vi "Finish.vi"   [LabVIEW 2012]
doc: "This VI is called just before exiting. It is expected to close I/O refnum, save collected data, etc."
uses:
  <vilib>/Rock Robotics/WPI/Joystick/WPI_JoystickGetSetRefNum.vi
  <vilib>/Rock Robotics/WPI/RobotDrive/WPI_RobotDriveGetSetRefNum.vi
types:
  T1 = typedef "WPI_CameraDevRef.ctl" = cluster{"Camera Address":string, "CameraStatus":errorcluster, "Acquire Image Notifier":refnum<notifier>}
  T2 = typedef "WPI_JoystickDevRef.ctl" = cluster{"Device":T3}
  T3 = typedef "WPI_JoystickDeviceEnum.ctl" = enum16{"USB 1", "USB 2", "USB 3", "USB 4", "Kinect 1", "Kinect 2"}
  T4 = typedef "WPI_RobotDriveDevRef.ctl" = cluster{"DevStatus":errorcluster, "Motors[]":T5[], "Square Inputs":bool, "Max Output":dbl, "Isochronous":bool}
  T5 = typedef "WPI_MotorControlDeviceRef.ctl" = cluster{"DeviceStatus":errorcluster, "Type":enum16{"PWM", "CAN"}, "PWM":cluster{"Digital Module":T6, "PWM Channel":T7, "DeadBand":T8}, "CAN":cluster{"Device Number":u8, "Control Mode":T9, "Semaphore":T10, "Max Vout":dbl}, "Invert":bool, "TransformRef":T11, "InvTransformRef":T11}
  T6 = typedef "FPGA_TypedefDigitalModule.ctl" = enum16{"Digital Module 1", "Digital Module 2"}
  T7 = typedef "FPGA_DIOPWMChannel.ctl" = enum8{"PWM 1", "PWM 2", "PWM 3", "PWM 4", "PWM 5", "PWM 6", "PWM 7", "PWM 8", "PWM 9", "PWM 10", "Invalid"}
  T8 = typedef "WPI_PWMDeadband.ctl" = cluster{"Name":string, "maxPositivePwm":i32, "minPositivePwm":i32, "centerPwm":i32, "maxNegativePwm":i32, "minNegativePwm":i32, "angularRange":u16}
  T9 = typedef "WPI_CANJaguar_ControlMode.ctl" = enum8{"Percent VBus", "Current", "Speed", "Position", "Voltage"}
  T10 = typedef "Semaphore RefNum" = refnum<k1>
  T11 = typedef "WPI_PWMTransform_ConPane.ctl" = refnum<vi>
  T12 = typedef "WPI_RelayDevRef.ctl" = cluster{"DevStatus":errorcluster, "Relay Channel":T13, "Digital Module":T6, "Relay Direction":T14}
  T13 = typedef "FPGA_DIORelayChannel.ctl" = enum8{"Relay 1", "Relay 2", "Relay 3", "Relay 4", "Relay 5", "Relay 6", "Relay 7", "Relay 8", "Invalid"}
  T14 = typedef "WPI_RelayDirection.ctl" = enum16{"Both directions", "Forward only", "Reverse only"}
  T15 = typedef "WPI_ServoDeviceRef.ctl" = cluster{"DeviceStatus":errorcluster, "Digital Module":T6, "PWM Channel":T7, "DeadBand":T8}
  T16 = typedef "WPI_I2CDevRef.ctl" = cluster{"DevStatus":errorcluster, "Digital Module":T6, "Device Address":u8}
  T17 = typedef "WPI_EncoderDevRef.ctl" = cluster{"DevStatus":errorcluster, "EncoderIndex":T18, "CounterIndex":T19, "DistancePerCount":dbl, "Decoding Type":T20}
  T18 = typedef "FPGA_EncoderIdx.ctl" = enum8{"Enc 0", "Enc 1", "Enc 2", "Enc 3", "Invalid"}
  T19 = typedef "FPGA_CounterCtrSystemIndex.ctl" = enum8{"Ctr 0", "Ctr 1", "Ctr 2", "Ctr 3", "Ctr 4", "Ctr 5", "Ctr 6", "Ctr 7", "Invalid"}
  T20 = typedef "WPI_EncoderType.ctl" = enum16{"1x", "2x", "4x"}
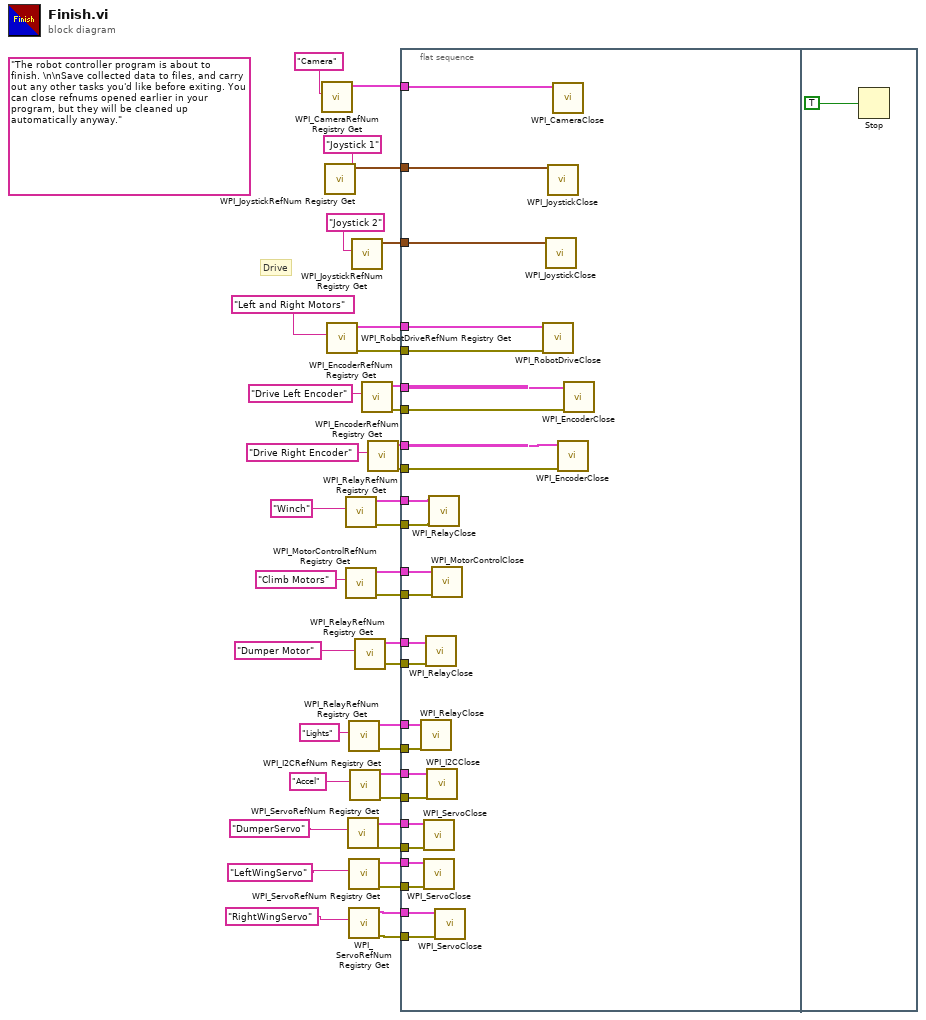
[diagram p0: block diagram]
diagram:
  (unwired) "The robot controller program is about to finish. \n\nSave collected data to files, and carry out any other tasks you'd like before exiting. You can close refnums opened earlier in your program, but they will be cleaned up automatically anyway."
  # "Drive"
  n1 = call <vilib>:"WPI_CameraRefNum Registry Get.vi"("refnum name"="Camera") -> ("CameraDevRef"=w35:T1)  [unwired: 1 in, 9 out]
  n2 = call <vilib>:"WPI_JoystickRefNum Registry Get.vi"("refnum name"="Joystick 1") -> ("JoystickDevRef"=w36:T2)  [unwired: 1 in, 9 out]
  n3 = call <vilib>:"WPI_RobotDriveRefNum Registry Get.vi"("refnum name"="Left and Right Motors") -> ("error out"=w10:errorcluster, "RobotDriveDevRef"=w37:T4)  [unwired: 1 in, 8 out]
  n4 = call <vilib>:"WPI_RelayRefNum Registry Get.vi"("refnum name"="Winch") -> ("error out"=w23:errorcluster, "RelayDevRef"=w24:T12)  [unwired: 9 in]
  n5 = call <vilib>:"WPI_MotorControlRefNum Registry Get.vi"("refnum name"="Climb Motors") -> ("error out"=w21:errorcluster, "MotorControlDevRef"=w22:T5)  [unwired: 9 in]
  n6 = call <vilib>:"WPI_ServoRefNum Registry Get.vi"("refnum name"="DumperServo") -> ("error out"=w4:errorcluster, "ServoDeviceRef"=w5:T15)  [unwired: 9 in]
  n7 = call <vilib>:"WPI_RelayRefNum Registry Get.vi"("refnum name"="Lights") -> ("error out"=w15:errorcluster, "RelayDevRef"=w16:T12)  [unwired: 9 in]
  n8 = call <vilib>:"WPI_ServoRefNum Registry Get.vi"("refnum name"="LeftWingServo") -> ("error out"=w7:errorcluster, "ServoDeviceRef"=w6:T15)  [unwired: 9 in]
  n9 = call <vilib>:"WPI_ServoRefNum Registry Get.vi"("refnum name"="RightWingServo") -> ("error out"=w8:errorcluster, "ServoDeviceRef"=w9:T15)  [unwired: 9 in]
  n10 = call <vilib>:"WPI_I2CRefNum Registry Get.vi"("refnum name"="Accel") -> ("error out"=w11:errorcluster, "I2CDevRef"=w12:T16)  [unwired: 9 in]
  n11 = call <vilib>:"WPI_JoystickRefNum Registry Get.vi"("refnum name"="Joystick 2") -> ("JoystickDevRef"=w32:T2)  [unwired: 1 in, 9 out]
  n12 = call <vilib>:"WPI_RelayRefNum Registry Get.vi"("refnum name"="Dumper Motor") -> ("error out"=w17:errorcluster, "RelayDevRef"=w18:T12)  [unwired: 9 in]
  n13 = call <vilib>:"WPI_EncoderRefNum Registry Get.vi"("refnum name"="Drive Left Encoder") -> ("error out"=w28:errorcluster, "EncoderDevRef"=w29:T17)  [unwired: 9 in]
  n14 = call <vilib>:"WPI_EncoderRefNum Registry Get.vi"("refnum name"="Drive Right Encoder") -> ("error out"=w26:errorcluster, "EncoderDevRef"=w27:T17)  [unwired: 9 in]
  n15 = flat-sequence {
    tunnel: w37 -> [w64]
    tunnel: w36 -> [w63]
    tunnel: w35 -> [w62]
    tunnel: w32 -> [w61]
    tunnel: w29 -> [w60]
    tunnel: w28 -> [w59]
    tunnel: w27 -> [w58]
    tunnel: w26 -> [w57]
    tunnel: w24 -> [w56]
    tunnel: w23 -> [w55]
    tunnel: w22 -> [w54]
    tunnel: w21 -> [w53]
    tunnel: w18 -> [w52]
    tunnel: w17 -> [w51]
    tunnel: w16 -> [w50]
    tunnel: w15 -> [w49]
    tunnel: w12 -> [w47]
    tunnel: w11 -> [w48]
    tunnel: w10 -> [w46]
    tunnel: w9 -> [w45]
    tunnel: w8 -> [w44]
    tunnel: w7 -> [w43]
    tunnel: w6 -> [w42]
    tunnel: w5 -> [w41]
    tunnel: w4 -> [w40]
    frame #0 {
      n16 = call <vilib>:"WPI_RelayClose.vi"("error in (no error)"=w49, "RelayDevRef"=w50) -> ()  [unwired: 9 in, 1 out]
      n17 = call <vilib>:"WPI_ServoClose.vi"("error in (no error)"=w40, "MotorControlDevRef"=w41) -> ()  [unwired: 9 in, 1 out]
      n18 = call <vilib>:"WPI_ServoClose.vi"("error in (no error)"=w43, "MotorControlDevRef"=w42) -> ()  [unwired: 9 in, 1 out]
      n19 = call <vilib>:"WPI_RelayClose.vi"("error in (no error)"=w51, "RelayDevRef"=w52) -> ()  [unwired: 9 in, 1 out]
      n20 = call <vilib>:"WPI_I2CClose.vi"("error in (no error)"=w48, "I2CDevRef"=w47) -> ()  [unwired: 9 in, 1 out]
      n21 = call <vilib>:"WPI_RelayClose.vi"("error in (no error)"=w55, "RelayDevRef"=w56) -> ()  [unwired: 9 in, 1 out]
      n22 = call <vilib>:"WPI_MotorControlClose.vi"("error in (no error)"=w53, "MotorControlDevRef"=w54) -> ()  [unwired: 9 in, 1 out]
      n23 = call <vilib>:"WPI_ServoClose.vi"("error in (no error)"=w44, "MotorControlDevRef"=w45) -> ()  [unwired: 9 in, 1 out]
      n24 = call <vilib>:"WPI_RobotDriveClose.vi"("error in (no error)"=w46, "RobotDriveDevRef"=w64) -> ()  [unwired: 10 out]
      n25 = call <vilib>:"WPI_JoystickClose.vi"("JoystickDevRef"=w61) -> ()  [unwired: 11 out]
      n26 = call <vilib>:"WPI_JoystickClose.vi"("JoystickDevRef"=w63) -> ()  [unwired: 11 out]
      n27 = call <vilib>:"WPI_CameraClose.vi"("CameraDevRef"=w62) -> ()  [unwired: 1 in, 10 out]
      n28 = call <vilib>:"WPI_EncoderClose.vi"("error in (no error)"=w57, "EncoderDevRef"=w58) -> ()  [unwired: 9 in, 1 out]
      n29 = call <vilib>:"WPI_EncoderClose.vi"("error in (no error)"=w59, "EncoderDevRef"=w60) -> ()  [unwired: 9 in, 1 out]
    }
    frame #1 {
      n30 = Stop(stop? (T)=TRUE ("Quit")) -> ()
    }
  }
